vi "Write to File.vi"(8 "error in":errorcluster, 10 "File Actor In":refnum<class "File Actor.lvclass">, 11 "Exe Write Main in":refnum<class "Exe Write PAS Waveforms.lvclass">) -> (0 "error out":errorcluster, 2 "File Actor Out":refnum<class "File Actor.lvclass">)   [LabVIEW 2018, in "Controller.lvlib" / "Exe Write PAS Waveforms.lvclass"]
doc: "In this command, we pole the MAP DVR which contains all of the data that is to be written to file...."
uses:
  Exe Write PAS Waveforms.lvclass
  File Actor/File Actor.lvclass
  C:/Users/Labview/Documents/exscalabar_server/SuperActor/SuperActor.lvclass
  reusable/Data/Data.lvclass
  SuperActor/SuperActor.lvclass/SuperActor.ctl
  File Actor/File Actor.lvclass/File Actor.ctl
  Exe Write PAS Waveforms.lvclass/Exe Write PAS Waveforms.ctl
  reusable/PAS/Data/Main/PAS Data.lvclass
  C:/Users/Labview/Documents/exscalabar_server/reusable/Data/Data.lvclass
  SuperActor/Read Log Session.vi
  File Actor/Read File DVR.vi
  reusable/Data/Read measTime.vi
  reusable/PAS/Data/Main/Read CellData.vi
  reusable/PAS/Data/Cell/Read timeData.vi
  reusable/PAS/Data/Cell/Read lasDiodeData.vi
  <userlib>/_Session Fwk/Session - Root.lvclass
  reusable/PAS/Data/Cell/PAS Cell Data.lvclass
  reusable/Session APIs/Session Log/System Log.lvclass
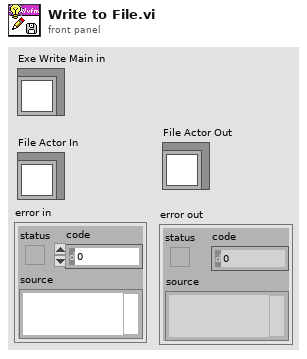
[diagram p1: front panel]
types:
  T1 = typedef "Session - Root.lvclass/Session Handle.ctl" = refnum<data-value>
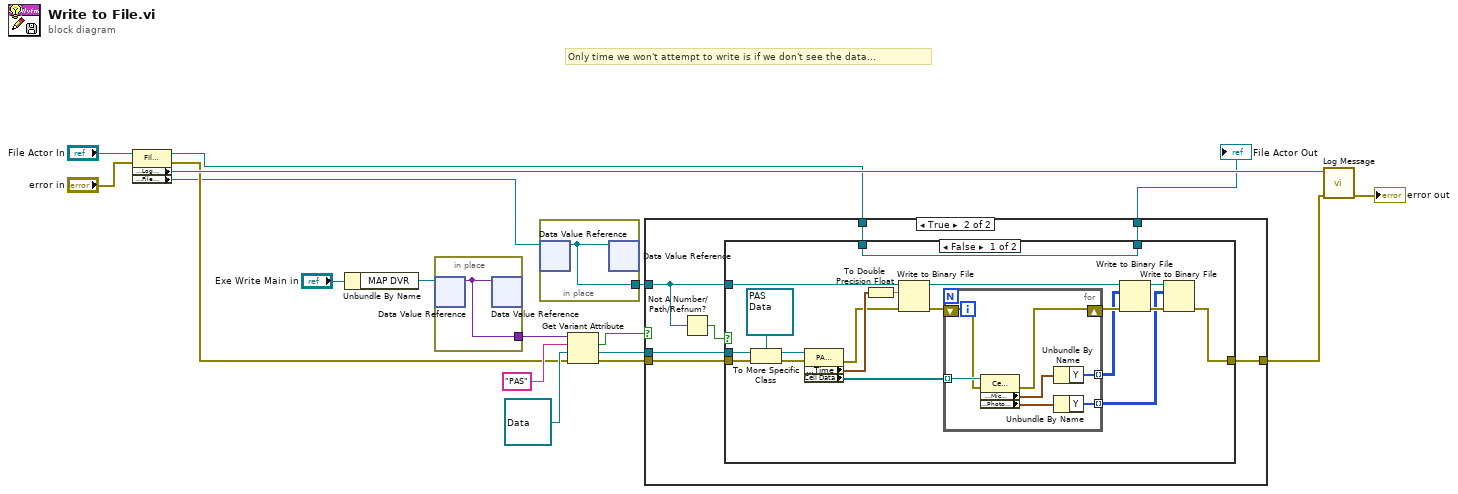
[diagram p0: block diagram]
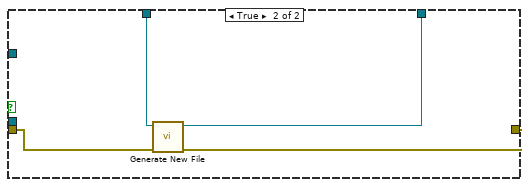
[diagram p3: hidden frame]
diagram:
  # "Only time we won't attempt to write is if we don't see the data..."
  n1 = property class="File Actor"(reference="File Actor In", error in="error in") -> (reference out=w2:refnum<class "File Actor.lvclass">, error out=w4:errorcluster, "Accessors:Log Session"=w12:T1, "Accessors:File DVR"=w3:refnum<data-value>)
  n2 = Unbundle By Name("Exe Write Main in") -> ("MAP DVR"=w14:refnum<data-value>)
  n3 = in-place {
    in-place-border: [w19] -> w13
    n4 = in-place-dvr #1(w14) -> (w19:variant)  [unwired: 1 out]
    n5 = in-place-dvr #1(w19) -> ()  [unwired: 2 out]
  }
  n6 = in-place {
    in-place-border: [w20] -> w17
    n7 = in-place-dvr #2(w3) -> (w20:refnum<file>)  [unwired: 1 out]
    n8 = in-place-dvr #2(w20) -> ()  [unwired: 2 out]
  }
  n9 = Get Variant Attribute(Variant=w13, name="PAS", default value (empty Variant)=refnum<class "Data.lvclass"> refnum ("Base Data Lib:Data"), error in=w4) -> (found=w6:bool, value=w7:refnum<class "Data.lvclass">, error out=w5:errorcluster)  [unwired: 1 out]
  n10 = case shown="True" w6 {
    tunnel: [w22 w27] -> w11
    tunnel: w17 -> [_ w25]
    tunnel: w7 -> [_ w29]
    tunnel: w5 -> [w22 w28]
    tunnel: w2 -> [w21 w24]
    tunnel: [w21 w23] -> w1
    frame False {
    }
    frame True {
      n11 = Not A Number/Path/Refnum?(number/path/refnum=w25) -> (NaN/Path/Refnum?=w26:bool)
      n12 = case shown="False" w26 {
        tunnel: w29 -> [w48 _]
        tunnel: w25 -> [w42 _]
        tunnel: w28 -> [w40 w56]
        tunnel: [w31 w57] -> w27
        tunnel: w24 -> [w30 w59]
        tunnel: [w30 w58] -> w23
        frame False {
          n13 = To More Specific Class(target class=refnum<class "PAS Data.lvclass"> refnum ("PAS Library.lvlib:PAS Data"), reference=w48, error in=w40) -> (specific class reference=w46:refnum<class "PAS Data.lvclass">, error out=w39:errorcluster)
          n14 = property class="PAS Data"(reference=w46, error in=w39) -> (error out=w38:errorcluster, "Accessors:Time"=w44:timestamp, "Cell Data"=w45:refnum<class "PAS Cell Data.lvclass">[])  [unwired: 1 out]
          n15 = To Double Precision Float(number=w44) -> (double precision float=w43:dbl)
          n16 = Write to Binary File(file (use dialog)=w42, data=w43, error in=w38) -> (refnum out=w36:refnum<file>, error out=w41:errorcluster)  [unwired: 3 in, 1 out]
          n17 = for {
            tunnel: w45 -> [w55] mode=indexing
            shift-right: [w51] -> w37
            shift-left: w41 -> [w54]
            tunnel: [w50] -> w35 mode=indexing
            tunnel: [w49] -> w32 mode=indexing
            n18 = property class="Cell Data"(reference=w55, error in=w54) -> (error out=w51:errorcluster, "Accessors:Mic Time"=w53:waveform(i16), "Accessors:Photodiode"=w52:waveform(i16))  [unwired: 1 out]
            n19 = Unbundle By Name(w53) -> ("Y"=w50:i16[])
            n20 = Unbundle By Name(w52) -> ("Y"=w49:i16[])
          }
          n21 = Write to Binary File(file (use dialog)=w36, data=w35, error in=w37) -> (refnum out=w34:refnum<file>, error out=w33:errorcluster)  [unwired: 3 in, 1 out]
          n22 = Write to Binary File(file (use dialog)=w34, data=w32, error in=w33) -> (error out=w31:errorcluster)  [unwired: 3 in, 2 out]
        }
        frame True {
          n23 = call "Generate New File.vi"("error in"=w56, "File Actor in"=w59) -> ("error out"=w57:errorcluster, "File Actor out"=w58:refnum<class "File Actor.lvclass">)  [unwired: 8 in]
        }
      }
    }
  }
  "File Actor Out" <- w1
  n24 = call "Log Message.vi"("error in"=w11, "session in"=w12) -> ("error out"=→"error out":errorcluster)  [unwired: 8 in, 1 out]
